vi "Connect.vi"(8 "error in (no error)":errorcluster, 11 "reference in":refnum<class "Camera_IMAQdx.lvclass">) -> (0 "error out":errorcluster, 3 "reference out":refnum<class "Camera_IMAQdx.lvclass">)   [LabVIEW 2017, in "Camera_IMAQdx.lvclass"]
doc: "Connects to the IMAQ camera with the configured interface name. Returns error if connection unsuccessful."
uses:
  Camera_IMAQdx.lvclass
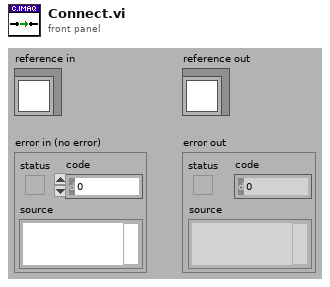
[diagram p1: front panel]
types:
  T1 = typedef "Camera_IMAQdx.lvclass/Configuration--Cluster.ctl" = cluster{"Camera Interface Name":string, "Number of Buffers":u32, "Image Name":string, "Image Type":T2}
  T2 = typedef "Image Type" = u32
  T3 = typedef "IMAQdx.ctl" = refnum<k21>
  T4 = typedef "IMAQ Image.ctl" = refnum<image>
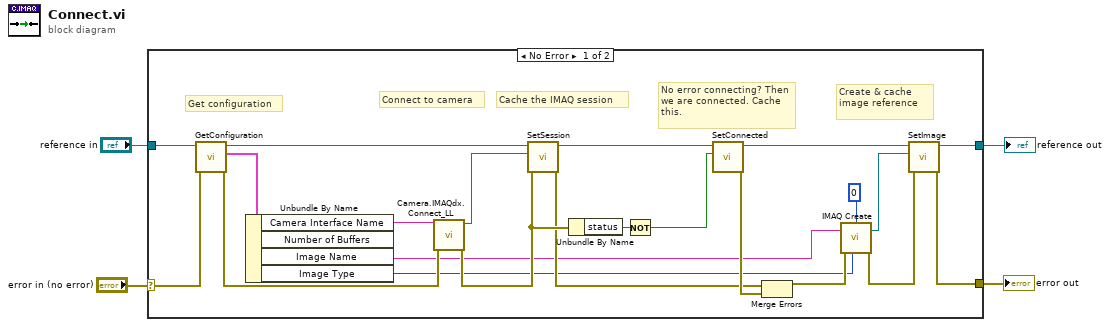
[diagram p0: block diagram]
diagram:
  n1 = case shown="No Error" "error in (no error)" {
    selector: "error in (no error)" -> [w22 w28]
    tunnel: [w7 w28] -> w3
    tunnel: [w10 w27] -> w1
    tunnel: "reference in" -> [w26 w27]
    frame No Error {
      # "Create & cache image reference"
      # "No error connecting? Then we are connected. Cache this."
      # "Cache the IMAQ session"
      # "Connect to camera"
      # "Get configuration"
      n2 = call-dynamic "GetConfiguration.vi"("error in (no error)"=w22, "reference in"=w26) -> ("error out"=w21:errorcluster, "Configuration"=w24:T1, "reference out"=w25:refnum<class "Camera_IMAQdx.lvclass">)  [unwired: 7 in]
      n3 = Unbundle By Name(w24) -> ("Camera Interface Name"=w23:string, "Image Name"=w13:string, "Image Type"=w6:T2)  [unwired: 1 out]
      n4 = call "Camera.IMAQdx.Connect_LL.vi"("Error In"=w21, "Interface"=w23) -> ("Error Out"=w17:errorcluster, "Session Out"=w20:T3)  [unwired: 8 in]
      n5 = call "SetSession.vi"("error in (no error)"=w17, "Session"=w20, "reference in"=w25) -> ("error out"=w15:errorcluster, "reference out"=w18:refnum<class "Camera_IMAQdx.lvclass">)  [unwired: 7 in]
      n6 = Unbundle By Name(w17) -> ("status"=w16:bool)
      n7 = Not(x=w16) -> (.not. x?=w14:bool)
      n8 = call "SetConnected.vi"("Connected"=w14, "reference in"=w18) -> ("error out"=w19:errorcluster, "reference out"=w11:refnum<class "Camera_IMAQdx.lvclass">)  [unwired: 8 in]
      n9 = Merge Errors(w15, w19) -> (w9:errorcluster)
      n10 = call "IMAQ Create"("Border Size"=0, "Image Name"=w13, "Image Type"=w6, "error in (no error)"=w9) -> ("New Image"=w12:T4, "error out"=w8:errorcluster)  [unwired: 1 out]
      n11 = call "SetImage.vi"("error in (no error)"=w8, "Image"=w12, "reference in"=w11) -> ("error out"=w7:errorcluster, "reference out"=w10:refnum<class "Camera_IMAQdx.lvclass">)  [unwired: 7 in]
    }
    frame Error {
    }
  }
  "error out" <- w3
  "reference out" <- w1
